vi "_Set Test Path.vi"(8 "error in (no error)":errorcluster, 10 "Path":path, 11 "VI in":refnum<vi>) -> (0 "error out":errorcluster, 3 "VI out":refnum<vi>)   [LabVIEW 2020]
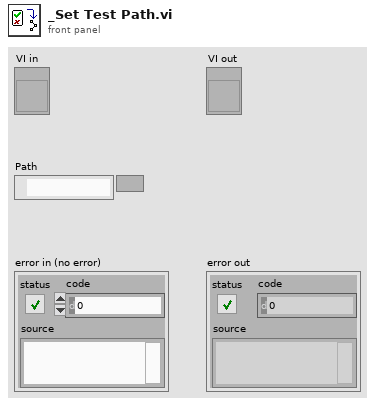
[diagram p1: front panel]
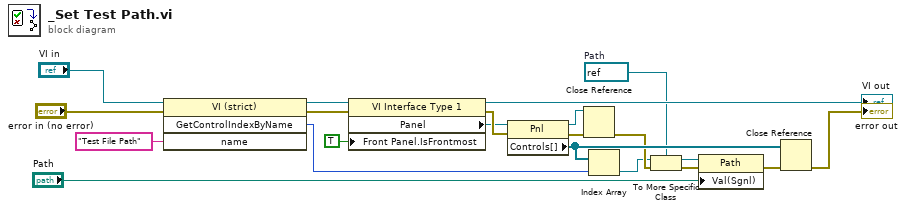
[diagram p0: block diagram]
diagram:
  w7 = refnum<vi> refnum  # Path
  n1 = invoke class="VI (strict)" method="GetControlIndexByName"(reference="VI in", error in="error in (no error)", "name"="Test File Path" ("Control Name")) -> (reference out=w4:refnum<vi>, error out=w13:errorcluster, "GetControlIndexByName"=w6:i32)  [unwired: 1 in, 1 out]
  n2 = property class="VI Interface Type 1"(reference=w4, error in=w13, "Front Panel.IsFrontmost"=TRUE ("Front Panel Window:Is Frontmost")) -> (reference out=→"VI out":refnum<vi>, error out=w12:errorcluster, "Panel"=w3:refnum<vi>)
  n3 = property class="Pnl"(reference=w3, error in=w12) -> (reference out=w16:refnum<vi>, error out=w11:errorcluster, "Controls[]"=w19:refnum<vi>[])
  n4 = Close Reference(reference=w16, error in (no error)=w11) -> (error out=w15:errorcluster)
  n5 = Index Array(array=w19, index=w6) -> (element=w9:refnum<vi>)
  n6 = To More Specific Class(target class=w7, reference=w9, error in=w15) -> (specific class reference=w8:refnum<vi>, error out=w10:errorcluster)
  n7 = property class="Path"(reference=w8, error in=w10, "Val(Sgnl)"="Path") -> (error out=w14:errorcluster)  [unwired: 1 out]
  n8 = Close Reference(reference=w19, error in (no error)=w14) -> (error out=→"error out":errorcluster)
